vi "SVN_CleanAllUnversioned.vi"(8 "error in (no error)":errorcluster, 10 "Path":string) -> (0 "error out":errorcluster, 1 "command":string, 2 "standard output":string, 3 "standard error":string)   [LabVIEW 2017]
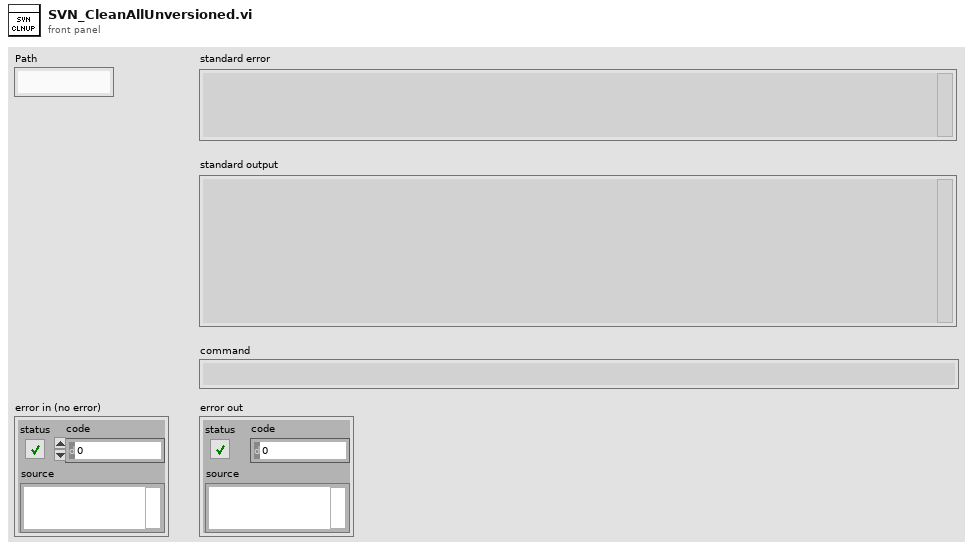
[diagram p1: front panel]
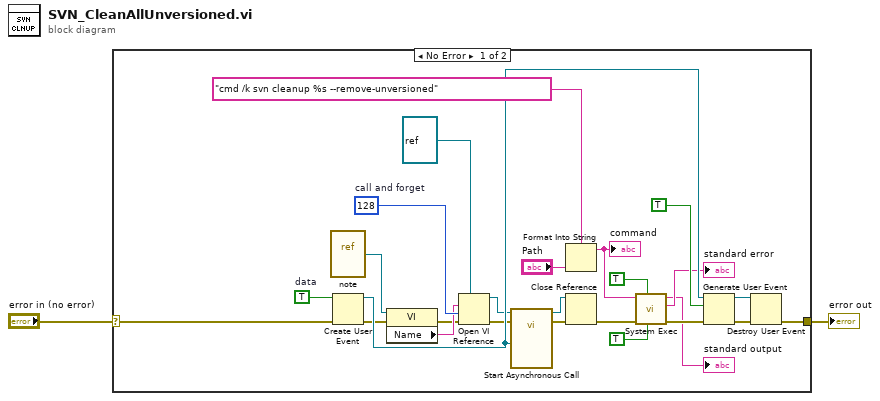
[diagram p0: block diagram]
diagram:
  n1 = case shown="No Error" "error in (no error)" {
    selector: "error in (no error)" -> [w21 w29]
    tunnel: [w23 w29] -> w2
    frame No Error {
      w24 = TRUE  # data
      w18 = 128  # call and forget
      n2 = vi-ref "note.vi"() -> (w19:refnum<vi>)
      n3 = Create User Event(user event datatype=w24, error in=w21) -> (user event=w25:refnum<user-event>, error out=w20:errorcluster)
      n4 = property class="VI"(reference=w19, error in=w20) -> (error out=w11:errorcluster, "Name"=w12:string)  [unwired: 1 out]
      n5 = Open VI Reference(type specifier VI Refnum (for type only)=refnum<vi> refnum, vi path=w12, options=w18, error in (no error)=w11) -> (vi reference=w16:refnum<vi>, error out=w15:errorcluster)  [unwired: 2 in]
      n6 = call-by-ref "Start Asynchronous Call"(reference=w16, error in=w15, "user event"=w25) -> (reference out=w13:refnum<vi>, error out=w14:errorcluster)  [unwired: 11 in]
      n7 = Format Into String(format string="cmd /k svn cleanup %s --remove-unversioned", "Path") -> (resulting string=w8:string)  [unwired: 2 in, 1 out]
      "command" <- w8
      n8 = Close Reference(reference=w13, error in (no error)=w14) -> (error out=w27:errorcluster)
      n9 = call <vilib>:"System Exec.vi"("run minimized? (F)"=TRUE, "wait until completion? (T)"=TRUE, "error in (no error)"=w27, "command line"=w8) -> ("error out"=w22:errorcluster, "standard error"=→"standard error":string, "standard output"=→"standard output":string)  [unwired: 4 in, 1 out]
      n10 = Generate User Event(user event=w25, event data cluster=TRUE ("event data"), error in=w22) -> (user event out=w28:refnum<user-event>, error out=w4:errorcluster)  [unwired: 1 in]
      n11 = Destroy User Event(user event=w28, error in=w4) -> (error out=w23:errorcluster)
    }
    frame Error {
    }
  }
  "error out" <- w2
